vi "Matrix Access.vi"() -> ()   [LabVIEW 2020]
panel:
  out "error out":errorcluster
  out "Intensity Graph":dbl[][](graph)
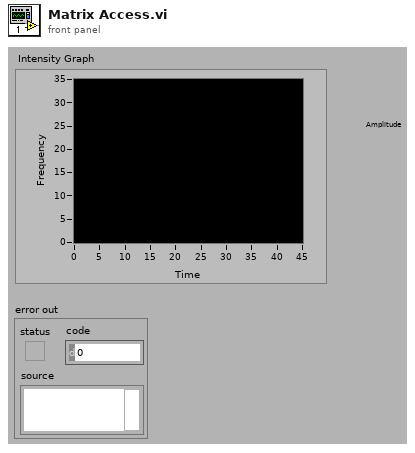
[diagram p1: front panel]
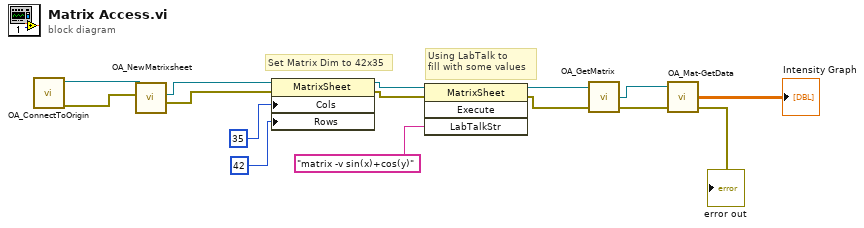
[diagram p0: block diagram]
diagram:
  # "Using LabTalk to\nfill with some values"
  # "Set Matrix Dim to 42x35"
  n1 = call "OA_ConnectToOrigin.vi"() -> ("error out"=w14:errorcluster, "Origin.IOApplication"=w15:refnum<k7>)  [unwired: 8 in]
  n2 = call "OA_NewMatrixsheet.vi"("error in (no error)"=w14, "Origin.IOApplication"=w15) -> ("error out"=w9:errorcluster, "Origin.MatrixSheet"=w13:refnum<k7>)  [unwired: 5 in, 1 out]
  n3 = property class="MatrixSheet"(reference=w13, error in=w9, "Cols"=35, "Rows"=42) -> (reference out=w10:refnum<k7>, error out=w8:errorcluster)
  n4 = invoke class="MatrixSheet" method="Execute"(reference=w10, error in=w8, "LabTalkStr"="matrix -v sin(x)+cos(y)") -> (reference out=w6:refnum<k7>, error out=w5:errorcluster)  [unwired: 1 in, 2 out]
  n5 = call "OA_GetMatrix.vi"("error in (no error)"=w5, "Origin.MatrixSheet"=w6) -> ("error out"=w3:errorcluster, "Matrix"=w4:refnum<k7>)  [unwired: 1 in, 1 out]
  n6 = call "OA_Mat-GetData.vi"("Origin.Matrix"=w4, "error in (no error)"=w3) -> ("Data"=→"Intensity Graph":dbl[][], "error out"=→"error out":errorcluster)  [unwired: 5 in, 1 out]
